vi "RAMP_scan_select-laser-lines.vi"(3 "error in":errorcluster, 5 "Laser lines array  IN":dbl[][](array[numeric])) -> (0 "Item Names":string[](array[string]), 1 "error out":errorcluster, 2 "Laser lines array":dbl[][](array[numeric]) format="%.2f")   [LabVIEW 2015]
panel:
  in  "Photobleaching time (s)":dbl
  in  "Laser application":dbl(ring)=1.0 items=["Select laser application", "merFISH", "Photobleaching"]
  in  "Remove":bool
  in  "stop":bool
  in  "Laser lines manager":i32(listbox)=-1
  in  "Add":bool
  in  "Laser line":dbl(ring) items=["Select laser line", "405 nm", "488 nm", "561 nm", "640 nm"]
  in  "Laser Power":dbl
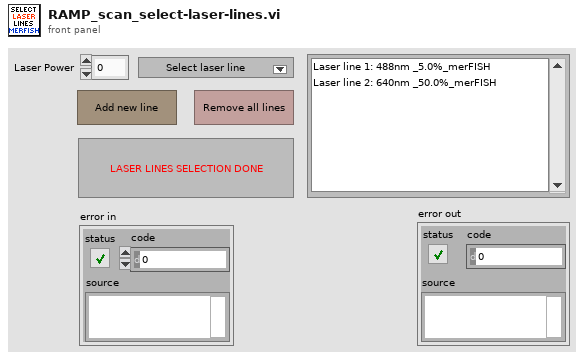
[diagram p1: front panel]
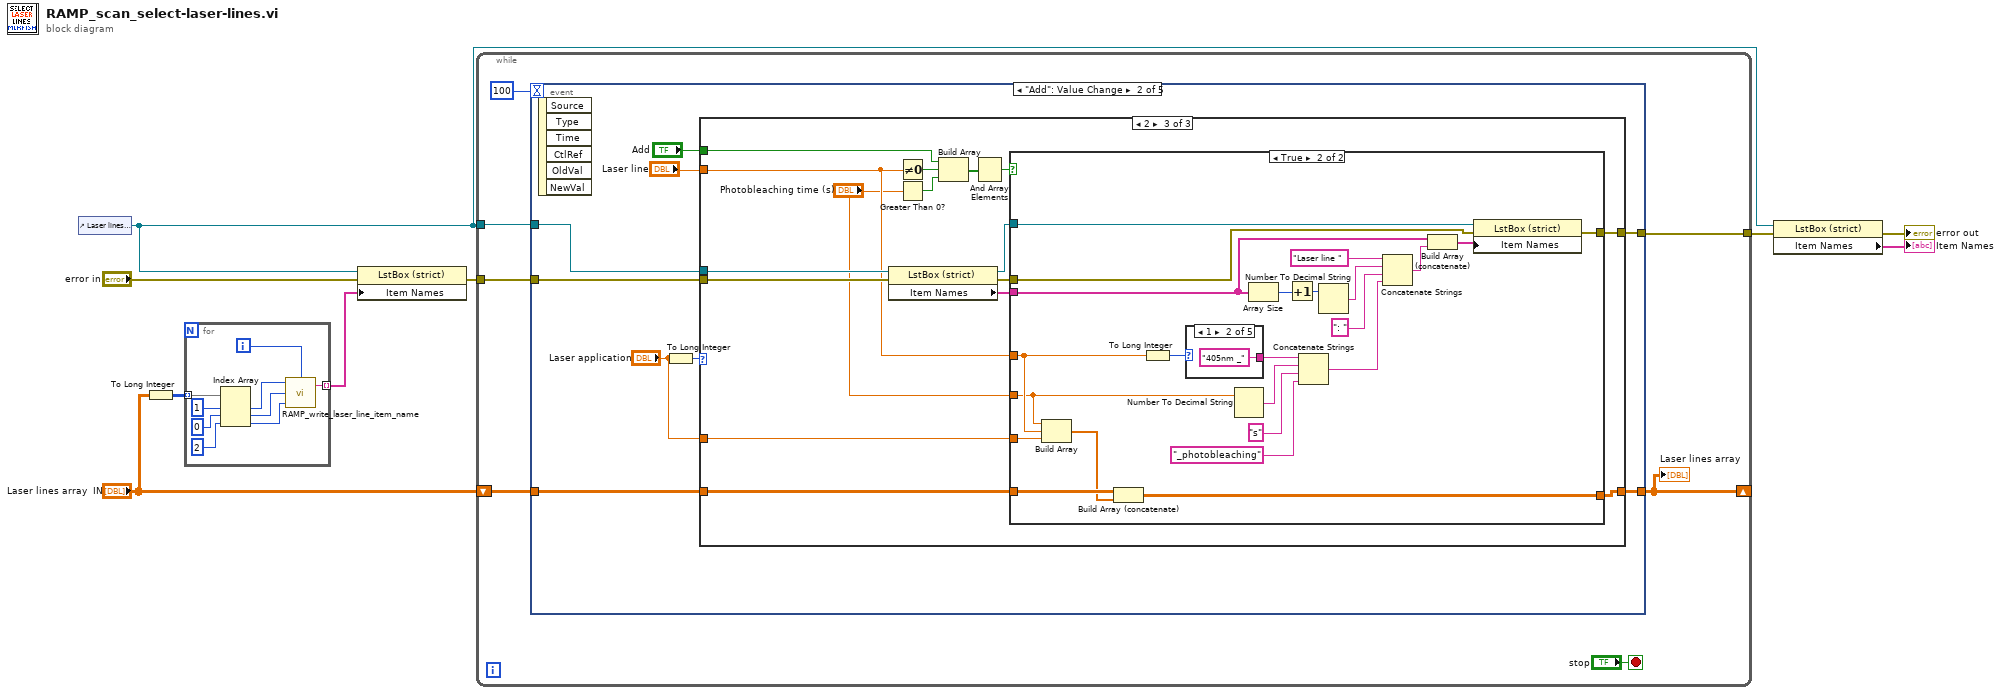
[diagram p0: block diagram]
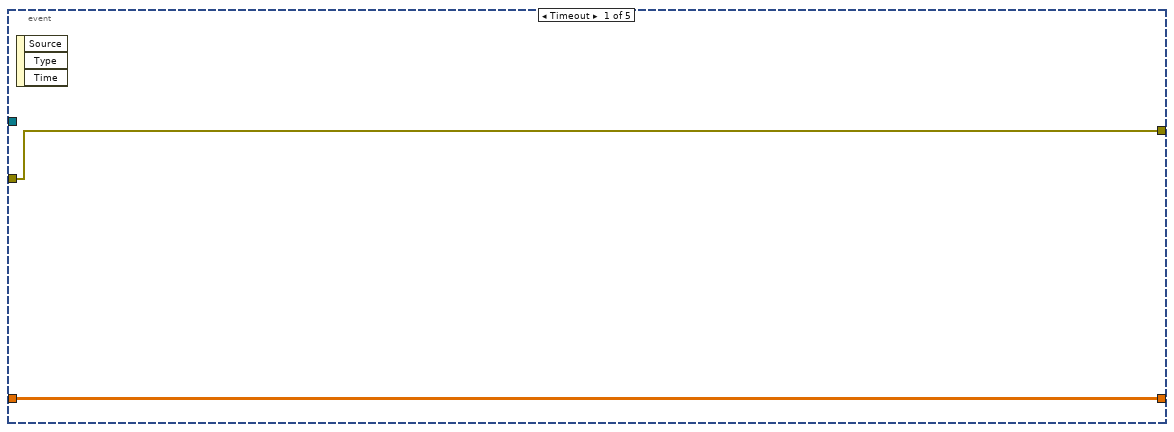
[diagram p2: hidden frame]
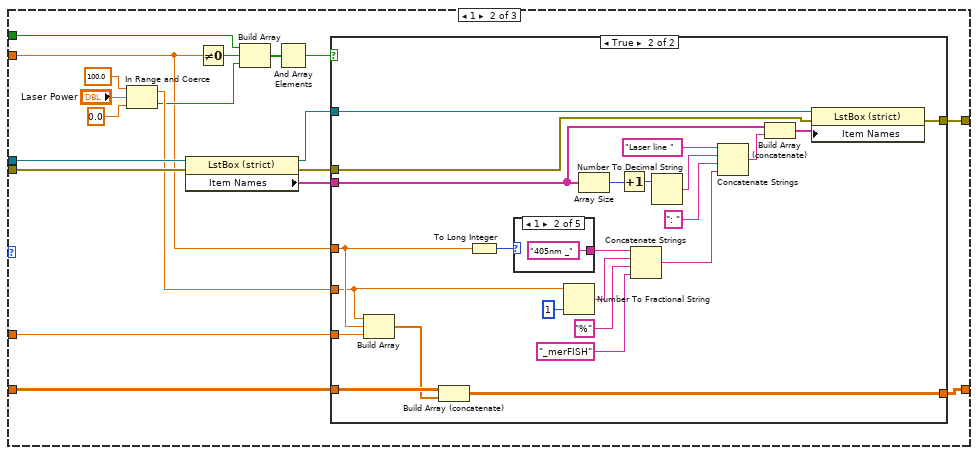
[diagram p4: hidden frame]
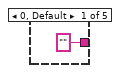
[diagram p6: hidden frame]
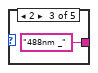
[diagram p7: hidden frame]
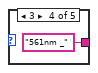
[diagram p8: hidden frame]
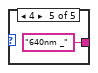
[diagram p9: hidden frame]
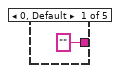
[diagram p11: hidden frame]
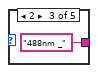
[diagram p12: hidden frame]
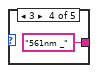
[diagram p13: hidden frame]
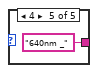
[diagram p14: hidden frame]
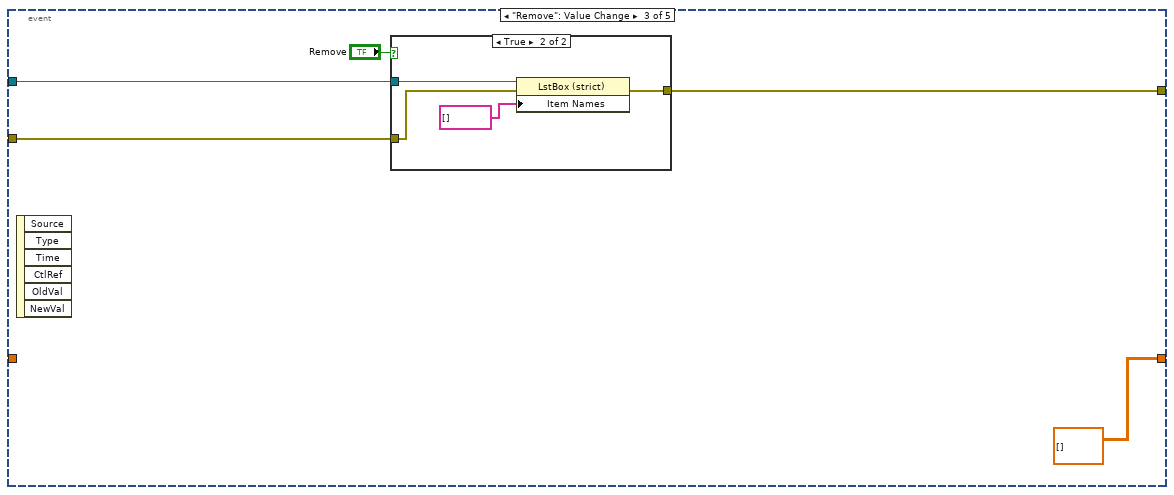
[diagram p15: hidden frame]
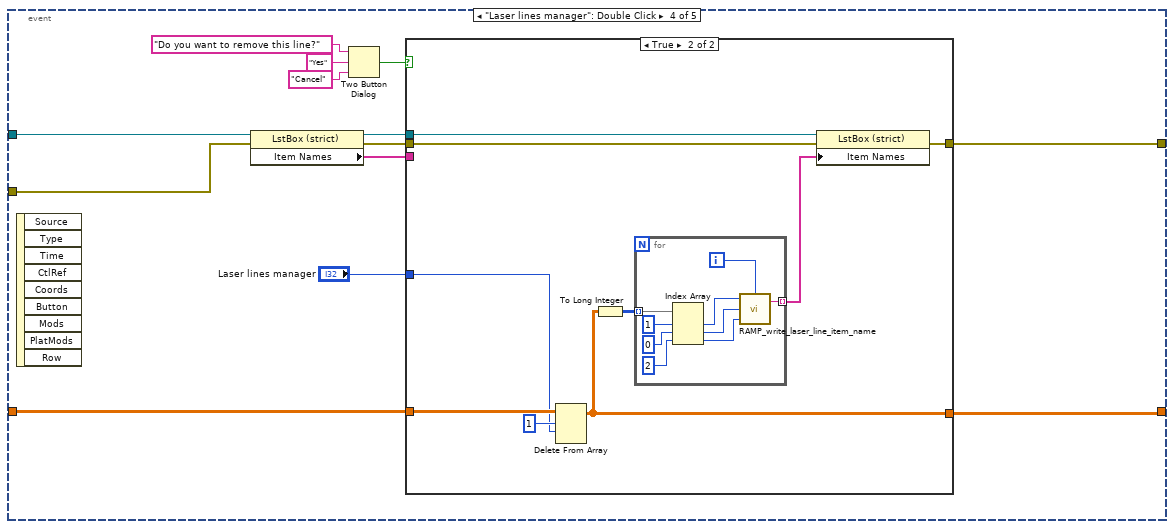
[diagram p17: hidden frame]
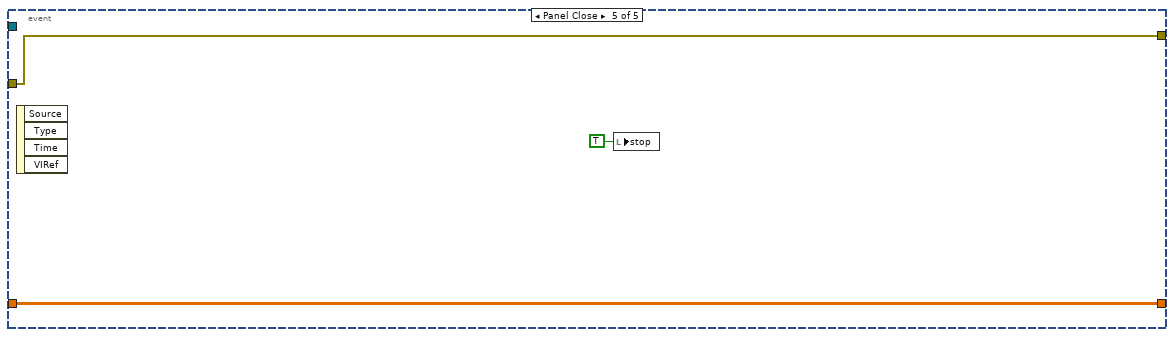
[diagram p19: hidden frame]
diagram:
  n1 = control-ref of="Laser lines manager"() -> (w3:refnum<vi>)
  n2 = To Long Integer(number="Laser lines array  IN") -> (32bit integer=w8:i32[][])
  n3 = for {
    tunnel: w8 -> [w17] mode=indexing
    tunnel: [w18] -> w4 mode=indexing
    i -> [w13]
    n4 = Index Array(array=w17, index #1=1 ("index"), index #2=0 ("index"), index #3=2 ("index")) -> (element #1=w12:i32, element #2=w11:i32, element #3=w10:i32)
    n5 = call "RAMP_write_laser_line_item_name.vi"("Laser line number"=w13, "Laser application"=w10, "Power or time"=w11, "Laser line"=w12) -> ("Item name"=w18:string)  [unwired: 1 in]
  }
  n6 = property class="LstBox (strict)"(reference=w3, error in="error in", "Item Names"=w4) -> (error out=w5:errorcluster)  [unwired: 1 out]
  n7 = while {
    tunnel: w3 -> [w23]
    tunnel: w5 -> [w20]
    tunnel: [w22] -> w9
    shift-right: [w19] -> _
    shift-left: "Laser lines array  IN" -> [w21]
    stop <- "stop" stop-if-true
    n8 = event shown="[1] \"Add\": Value Change" {
      selector: _ -> [_ _ _ _ _]
      dyn-events: _ -> [_ _ _ _ _]
      timeout: 100 -> [_ _ _ _ _]
      tunnel: w23 -> [_ w33 w139 w150 _]
      tunnel: w20 -> [w26 w34 w137 w148 w179]
      tunnel: [w26 w36 w136 w153 w179] -> w22
      tunnel: w21 -> [w27 w35 _ w152 w180]
      tunnel: [w27 w32 dbl[][] [] ("appended array") w145 w180] -> w19
      event Timeout {
        n9 = event-data() -> ()  [unwired: 1 in, 3 out]
      }
      event "Add": Value Change {
        n10 = event-data() -> ()  [unwired: 1 in, 6 out]
        n11 = To Long Integer(number="Laser application") -> (32bit integer=w31:i32)
        n12 = case shown="2" w31 {
          tunnel: [w38 w54 w101] -> w36
          tunnel: w35 -> [w37 w53 w100]
          tunnel: w34 -> [w38 w51 w98]
          tunnel: w33 -> [_ w50 w97]
          tunnel: [w37 w42 w94] -> w32
          tunnel: "Laser application" -> [_ w41 w93]
          tunnel: "Add" -> [_ w40 w92]
          tunnel: "Laser line" -> [_ w39 w91]
          frame 0, Default {
          }
          frame 1 {
            n13 = In Range and Coerce(upper limit=100.0, x="Laser Power", lower limit=0.0) -> (coerced(x)=w44:dbl, In Range?=w43:bool)
            n14 = property class="LstBox (strict)"(reference=w50, error in=w51) -> (reference out=w49:refnum<vi>, error out=w52:errorcluster, "Item Names"=w48:string[])
            n15 = Not Equal To 0?(x=w39) -> (x != 0?=w57:bool)
            n16 = Build Array(w40, w57, w43) -> (w56:bool[])
            n17 = And Array Elements(Boolean array=w56) -> (logical AND=w55:bool)
            n18 = case shown="True" w55 {
              tunnel: w49 -> [_ w79]
              tunnel: w39 -> [_ w71]
              tunnel: w44 -> [_ w64]
              tunnel: [w59 w72] -> w54
              tunnel: w52 -> [w59 w65]
              tunnel: w53 -> [w58 w70]
              tunnel: [w58 w68] -> w42
              tunnel: w48 -> [_ w66]
              tunnel: w41 -> [_ w61]
              frame False {
              }
              frame True {
                n19 = Build Array(w64, w71, w61) -> (w69:dbl[])
                n20 = Build Array (concatenate)(w70, w69) -> (w68:dbl[][])
                n21 = To Long Integer(number=w71) -> (32bit integer=w62:i32)
                n22 = case shown="1" w62 {
                  tunnel: ["" "405nm _" "488nm _" "561nm _" "640nm _"] -> w76
                  frame 0, Default {
                  }
                  frame 1 {
                  }
                  frame 2 {
                  }
                  frame 3 {
                  }
                  frame 4 {
                  }
                }
                n23 = Number To Fractional String(number=w64, precision (6)=i16 1) -> (F-format string=w75:string)  [unwired: 2 in]
                n24 = Array Size(array=w66) -> (size(s)=w78:i32)
                n25 = Increment(x=w78) -> (x+1=w82:i32)
                n26 = Concatenate Strings(w76, w75, "%" ("string"), "_merFISH") -> (w73:string)
                n27 = Number To Decimal String(number=w82) -> (decimal integer string=w81:string)  [unwired: 1 in]
                n28 = Concatenate Strings("Laser line " ("string"), w81, ": " ("string"), w73) -> (w80:string)
                n29 = Build Array (concatenate)(w66, w80) -> (w67:string[])
                n30 = property class="LstBox (strict)"(reference=w79, error in=w65, "Item Names"=w67) -> (error out=w72:errorcluster)  [unwired: 1 out]
              }
            }
          }
          frame 2 {
            n31 = property class="LstBox (strict)"(reference=w97, error in=w98) -> (reference out=w96:refnum<vi>, error out=w99:errorcluster, "Item Names"=w95:string[])
            n32 = Not Equal To 0?(x=w91) -> (x != 0?=w104:bool)
            n33 = Greater Than 0?(x="Photobleaching time (s)") -> (x > 0?=w89:bool)
            n34 = Build Array(w92, w104, w89) -> (w103:bool[])
            n35 = And Array Elements(Boolean array=w103) -> (logical AND=w102:bool)
            n36 = case shown="True" w102 {
              tunnel: w96 -> [_ w125]
              tunnel: w91 -> [_ w117]
              tunnel: "Photobleaching time (s)" -> [_ w110]
              tunnel: [w106 w118] -> w101
              tunnel: w99 -> [w106 w111]
              tunnel: w100 -> [w105 w116]
              tunnel: [w105 w114] -> w94
              tunnel: w95 -> [_ w112]
              tunnel: w93 -> [_ w107]
              frame False {
              }
              frame True {
                n37 = Build Array(w110, w117, w107) -> (w115:dbl[])
                n38 = Build Array (concatenate)(w116, w115) -> (w114:dbl[][])
                n39 = To Long Integer(number=w117) -> (32bit integer=w108:i32)
                n40 = case shown="1" w108 {
                  tunnel: ["" "405nm _" "488nm _" "561nm _" "640nm _"] -> w122
                  frame 0, Default {
                  }
                  frame 1 {
                  }
                  frame 2 {
                  }
                  frame 3 {
                  }
                  frame 4 {
                  }
                }
                n41 = Number To Decimal String(number=w110) -> (decimal integer string=w121:string)  [unwired: 1 in]
                n42 = Array Size(array=w112) -> (size(s)=w124:i32)
                n43 = Increment(x=w124) -> (x+1=w128:i32)
                n44 = Concatenate Strings(w122, w121, "s" ("string"), "_photobleaching") -> (w119:string)
                n45 = Number To Decimal String(number=w128) -> (decimal integer string=w127:string)  [unwired: 1 in]
                n46 = Concatenate Strings("Laser line " ("string"), w127, ": " ("string"), w119) -> (w126:string)
                n47 = Build Array (concatenate)(w112, w126) -> (w113:string[])
                n48 = property class="LstBox (strict)"(reference=w125, error in=w111, "Item Names"=w113) -> (error out=w118:errorcluster)  [unwired: 1 out]
              }
            }
          }
        }
      }
      event "Remove": Value Change {
        n49 = event-data() -> ()  [unwired: 1 in, 6 out]
        n50 = case shown="True" "Remove" {
          tunnel: w139 -> [_ w144]
          tunnel: w137 -> [w140 w143]
          tunnel: [w140 w142] -> w136
          frame False {
          }
          frame True {
            n51 = property class="LstBox (strict)"(reference=w144, error in=w143, "Item Names"=string[] []) -> (error out=w142:errorcluster)  [unwired: 1 out]
          }
        }
      }
      event "Laser lines manager": Double Click {
        n52 = event-data() -> ()  [unwired: 1 in, 9 out]
        n53 = property class="LstBox (strict)"(reference=w150, error in=w148) -> (reference out=w149:refnum<vi>, error out=w147:errorcluster, "Item Names"=w146:string[])
        n54 = Two Button Dialog(message="Do you want to remove this line?", 1:"Cancel" ("F button name (\"Cancel\")"), 2:"Yes" ("T button name (\"OK\")")) -> (T button?=w154:bool)
        n55 = case shown="True" w154 {
          tunnel: w149 -> [_ w163]
          tunnel: [w158 w168] -> w153
          tunnel: w152 -> [w159 w167]
          tunnel: [w159 w161] -> w145
          tunnel: "Laser lines manager" -> [_ w165]
          tunnel: w147 -> [w158 w164]
          tunnel: w146 -> [_ _]
          frame False {
          }
          frame True {
            n56 = Delete From Array(array=w167, length=1, index (row)=w165) -> (array with subset deleted=w161:dbl[][])  [unwired: 1 in, 1 out]
            n57 = To Long Integer(number=w161) -> (32bit integer=w160:i32[][])
            n58 = for {
              tunnel: w160 -> [w176] mode=indexing
              tunnel: [w177] -> w162 mode=indexing
              i -> [w172]
              n59 = Index Array(array=w176, index #1=1 ("index"), index #2=0 ("index"), index #3=2 ("index")) -> (element #1=w171:i32, element #2=w170:i32, element #3=w169:i32)
              n60 = call "RAMP_write_laser_line_item_name.vi"("Laser line number"=w172, "Laser application"=w169, "Power or time"=w170, "Laser line"=w171) -> ("Item name"=w177:string)  [unwired: 1 in]
            }
            n61 = property class="LstBox (strict)"(reference=w163, error in=w164, "Item Names"=w162) -> (error out=w168:errorcluster)  [unwired: 1 out]
          }
        }
      }
      event Panel Close {
        n62 = event-data() -> ()  [unwired: 1 in, 4 out]
        n63 = local write "stop"(TRUE ("stop")) -> ()
      }
    }
    "Laser lines array" <- w19
  }
  n64 = property class="LstBox (strict)"(reference=w3, error in=w9) -> (error out=→"error out":errorcluster, "Item Names"=→"Item Names":string[])  [unwired: 1 out]
